vi "ID Query.vi"(8 "error in":errorcluster, 10 "ID Query":bool, 11 "AcopianERP in":refnum<class "Acopian.lvclass">) -> (0 "error out":errorcluster, 3 "AcopianERP out":refnum<class "Acopian.lvclass">)   [LabVIEW 2019, in "Acopian.lvlib" / "Acopian.lvclass"]
uses:
  Library/Acopian.lvclass
  Library/Acopian.lvclass/Acopian.ctl
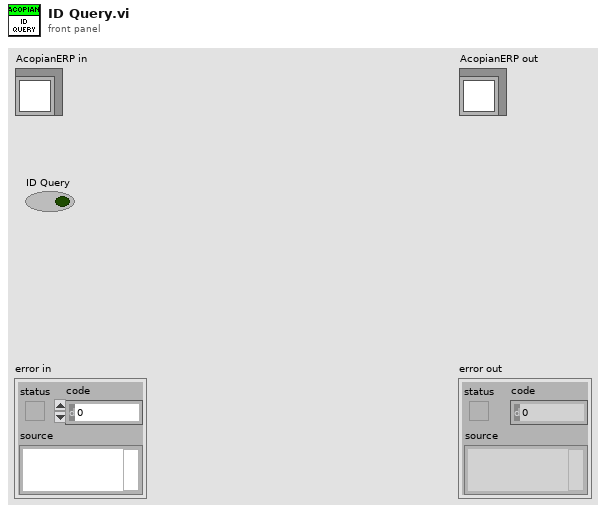
[diagram p1: front panel]
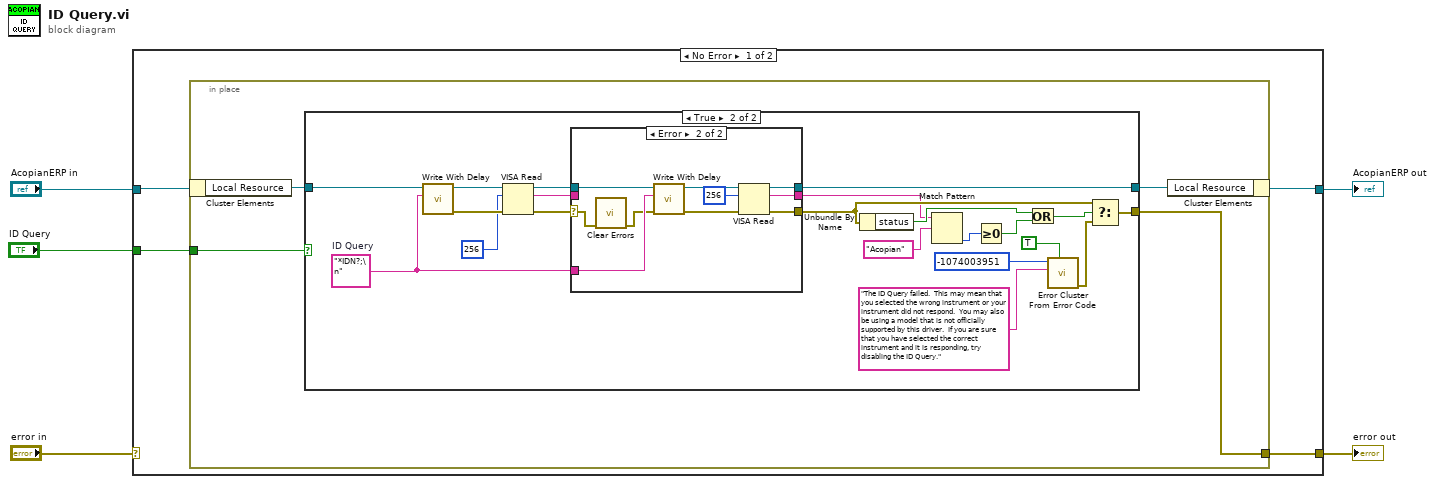
[diagram p0: block diagram]
diagram:
  n1 = case shown="No Error" "error in" {
    selector: "error in" -> [_ w50]
    tunnel: [w7 w50] -> w4
    tunnel: [w8 w49] -> w2
    tunnel: "AcopianERP in" -> [w9 w49]
    tunnel: "ID Query" -> [w6 _]
    frame No Error {
      n2 = in-place {
        in-place-border: [w11] -> w7
        in-place-border: w6 -> [w10]
        n3 = in-place-cluster #1(w9) -> ("Local Resource"=w13:refnum<visa-resource-name>)
        n4 = case shown="True" w10 {
          tunnel: [_ w35] -> w11
          tunnel: [w14 w19] -> w12
          tunnel: w13 -> [w14 w22]
          frame False {
          }
          frame True {
            w15 = "*IDN?;\n"  # ID Query
            n5 = call "Write With Delay.vi"("write buffer"=w15, "VISA resource name"=w22) -> ("error out"=w33:errorcluster, "VISA resource name out"=w34:refnum<visa-resource-name>)  [unwired: 8 in]
            n6 = VISA Read(VISA resource name=w34, byte count=u32 256, error in (no error)=w33) -> (VISA resource name out=w18:refnum<visa-resource-name>, read buffer=w16:string, error out=w21:errorcluster)  [unwired: 1 out]
            n7 = case shown="Error" w21 {
              selector: w21 -> [w37 w45]
              tunnel: [w37 w47] -> w20
              tunnel: [w38 w46] -> w19
              tunnel: w18 -> [w38 w43]
              tunnel: [w36 w44] -> w17
              tunnel: w16 -> [w36 _]
              tunnel: w15 -> [_ w42]
              frame No Error {
              }
              frame Error {
                n8 = call <vilib>:"Clear Errors.vi"("error in (no error)"=w45) -> ("error out"=w41:errorcluster)  [unwired: 5 in, 1 out]
                n9 = call "Write With Delay.vi"("error in"=w41, "write buffer"=w42, "VISA resource name"=w43) -> ("error out"=w40:errorcluster, "VISA resource name out"=w39:refnum<visa-resource-name>)  [unwired: 7 in]
                n10 = VISA Read(VISA resource name=w39, byte count=u32 256, error in (no error)=w40) -> (VISA resource name out=w46:refnum<visa-resource-name>, read buffer=w44:string, error out=w47:errorcluster)  [unwired: 1 out]
              }
            }
            n11 = Unbundle By Name(w20) -> ("status"=w25:bool)
            n12 = Match Pattern(string=w17, regular expression="Acopian") -> (offset past match=w26:i32)  [unwired: 1 in, 3 out]
            n13 = Greater Or Equal To 0?(x=w26) -> (x >= 0?=w24:bool)
            n14 = Or(x=w25, y=w24) -> (x .or. y?=w23:bool)
            n15 = call <vilib>:"Error Cluster From Error Code.vi"("show call chain? (False)"=TRUE, "error message (\"\")"="The ID Query failed.  This may mean that you selected the wrong instrument or your instrument did not respond.  You may also be using a model that is not officially supported by this driver.  If you are sure that you have selected the correct instrument and it is responding, try disabling the ID Query." ("Source (VI Name)"), "error code (0)"=-1074003951 ("Code")) -> ("error out"=w30:errorcluster)  [unwired: 6 in]
            n16 = Select(t=w20, s=w23, f=w30) -> (s? t:f=w35:errorcluster)
          }
        }
        n17 = in-place-cluster #1("Local Resource"=w12) -> (w8:refnum<class "Acopian.lvclass">)
      }
    }
    frame Error {
    }
  }
  "error out" <- w4
  "AcopianERP out" <- w2
